vi "LVP_compresion.vi"(11 "file path (dialog if empty)":path) -> (3 "file path out (Not A Path if cancelled)":path)   [LabVIEW 2012]
uses:
  <vilib>/Utility/file.llb/Read From Spreadsheet File (string).vi
  <vilib>/Utility/file.llb/Write To Spreadsheet File (string).vi
panel:
  out "all rows 2":string[][](array[string])
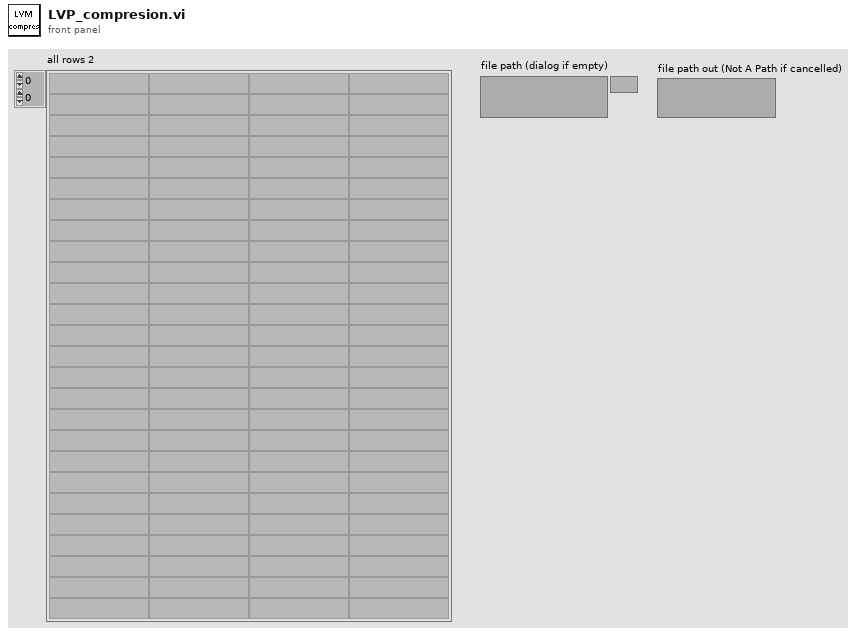
[diagram p1: front panel]
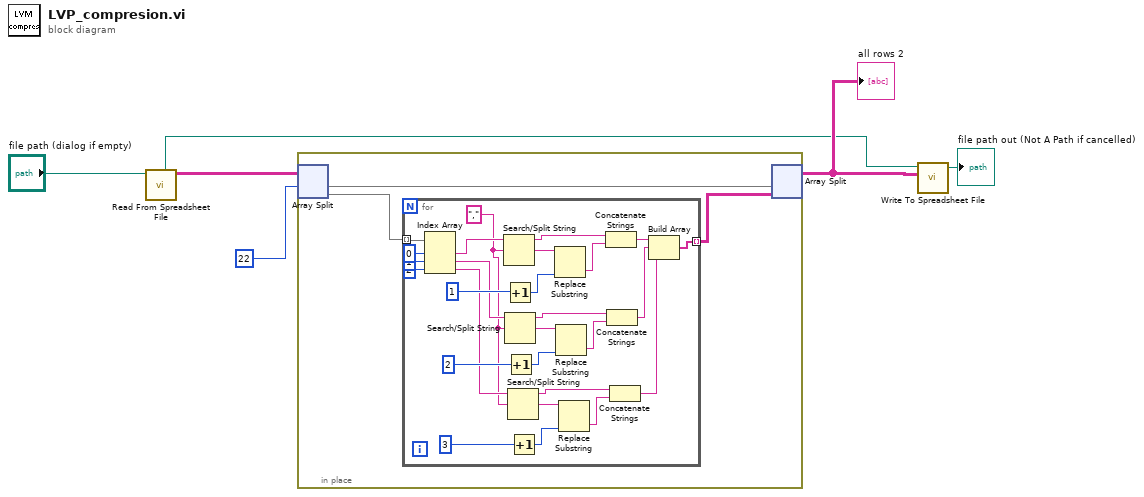
[diagram p0: block diagram]
diagram:
  n1 = call-poly <vilib>:"Read From Spreadsheet File.vi"("file path (dialog if empty)"="file path (dialog if empty)") -> ("all rows"=w6:string[][], "new file path (Not A Path if cancelled)"=w3:path)  [unwired: 6 in, 3 out]
  n2 = in-place {
    n3 = in-place-split #1(w6, 22 ("Numeric")) -> (w9:string[][], w8:string[][])
    n4 = for {
      tunnel: w8 -> [w31] mode=indexing
      tunnel: [w11] -> w7 mode=indexing
      w10 = "," ("search string/char (-)")
      n5 = Index Array(array=w31, index #1=0 ("index"), index #2=1 ("index"), index #3=2 ("index")) -> (element #1=w27:string, element #2=w21:string, element #3=w15:string)
      n6 = Search/Split String(string=w27, search string/char (-)=w10) -> (substring before match=w35:string, match + rest of string=w32:string)  [unwired: 1 in, 1 out]
      n7 = Increment(x=1 ("length (len. of substring)")) -> (x+1=w34:i32)
      n8 = Search/Split String(string=w21, search string/char (-)=w10) -> (substring before match=w23:string, match + rest of string=w26:string)  [unwired: 1 in, 1 out]
      n9 = Increment(x=2 ("length (len. of substring)")) -> (x+1=w24:i32)
      n10 = Search/Split String(string=w15, search string/char (-)=w10) -> (substring before match=w19:string, match + rest of string=w16:string)  [unwired: 1 in, 1 out]
      n11 = Increment(x=3 ("length (len. of substring)")) -> (x+1=w18:i32)
      n12 = Replace Substring(2:w34, 5:w32) -> (0:w36:string)  [unwired: 2 in, 1 out]
      n13 = Replace Substring(2:w24, 5:w26) -> (0:w22:string)  [unwired: 2 in, 1 out]
      n14 = Replace Substring(2:w18, 5:w16) -> (0:w20:string)  [unwired: 2 in, 1 out]
      n15 = Concatenate Strings(w35, w36) -> (w14:string)
      n16 = Concatenate Strings(w23, w22) -> (w13:string)
      n17 = Concatenate Strings(w19, w20) -> (w12:string)
      n18 = Build Array(w14, w13, w12) -> (w11:string[])
    }
    n19 = in-place-split #1(w9, w7) -> (w4:string[][])  [unwired: 1 out]
  }
  "all rows 2" <- w4
  n20 = call-poly <vilib>:"Write To Spreadsheet File.vi"("2D data"=w4, "file path (dialog if empty)"=w3) -> ("new file path (Not A Path if cancelled)"=→"file path out (Not A Path if cancelled)":path)  [unwired: 6 in]
